vi "Main.vi"() -> ()   [LabVIEW 2020]
uses:
  NI-9361 (C Series)/NI-9361 (C Series).lvclass
  C:/Users/Thomas/Documents/YouTube Videos/Interfaces/Interface HAL Example/C-Series/C-Series.lvclass
  NI-9421 (C Series)/NI-9421 (C Series).lvclass
  C:/Users/Thomas/Documents/YouTube Videos/Interfaces/Interface HAL Example/DIO/DIO.lvclass
  C-Series/C-Series.lvclass
  NI-6537 (PXIe)/NI-6537 (PXIe).lvclass
  C:/Users/Thomas/Documents/YouTube Videos/Interfaces/Interface HAL Example/PXIe/PXIe.lvclass
  PXIe/PXIe.lvclass
  Voltage Input/Voltage Input.lvclass
  NI-6115 (PXIe-6368)/NI-6368 (PXIe).lvclass
  C:/Users/Thomas/Documents/YouTube Videos/Interfaces/Interface HAL Example/Voltage Input/Voltage Input.lvclass
  C:/Users/Thomas/Documents/YouTube Videos/Interfaces/Interface HAL Example/DMM/Multifunction IO.lvclass
  NI-9381 (c series)/NI-9381 (c series).lvclass
  NI-9239 (C Series)/NI-9239 (C Series).lvclass
  PSU/AIO.lvclass
  Counter/Counter.lvclass
  DIO/DIO.lvclass
  Hardware/Instrument.lvclass
  DMM/Multifunction IO.lvclass
panel:
  in  "Select":bool
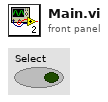
[diagram p1: front panel]
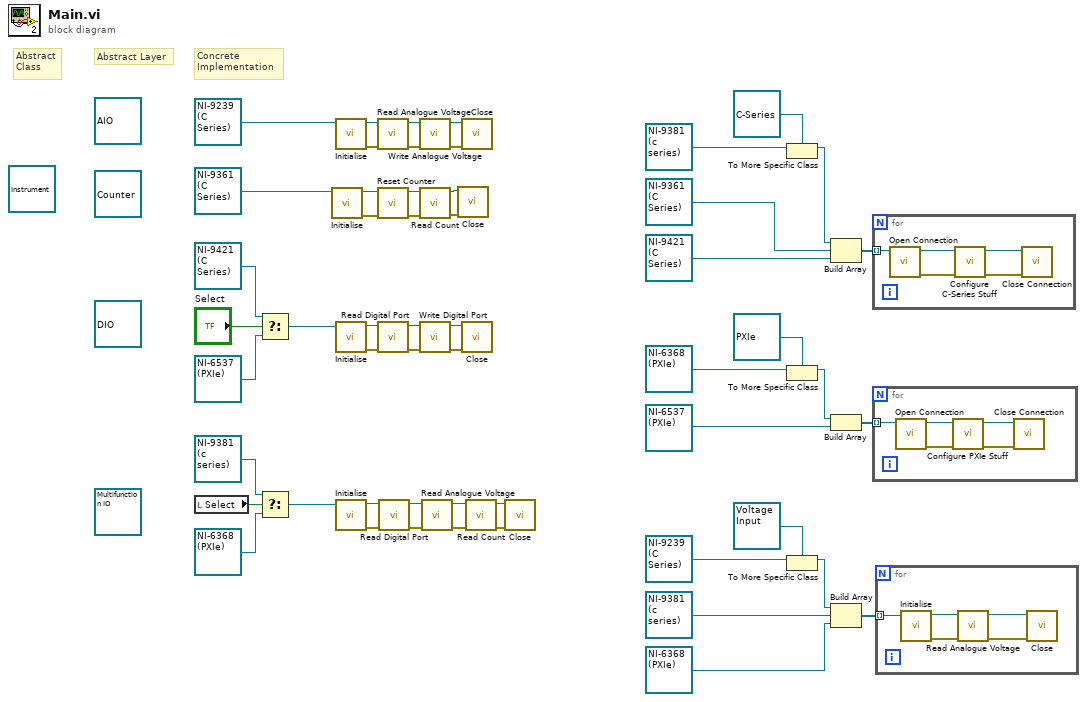
[diagram p0: block diagram]
diagram:
  (unwired) refnum<class "Multifunction IO.lvclass"> refnum ("Multifunction IO.lvclass")
  (unwired) refnum<class "Instrument.lvclass"> refnum ("Instrument.lvclass")
  (unwired) refnum<class "DIO.lvclass"> refnum ("DIO.lvclass")
  (unwired) refnum<class "Counter.lvclass"> refnum ("Counter.lvclass")
  (unwired) refnum<class "AIO.lvclass"> refnum ("AIO.lvclass")
  # "Concrete\nImplementation"
  # "Abstract\nClass"
  # "Abstract Layer"
  n1 = local read "Select"() -> (w34:bool)
  n2 = Select(t=refnum<class "NI-9421 (C Series).lvclass"> refnum ("NI-9421 (C Series).lvclass"), s="Select", f=refnum<class "NI-6537 (PXIe).lvclass"> refnum ("NI-6537 (PXIe).lvclass")) -> (s? t:f=w36:refnum<class "DIO.lvclass">)
  n3 = Select(t=refnum<class "NI-9381 (c series).lvclass"> refnum ("NI-9381 (c series).lvclass"), s=w34, f=refnum<class "NI-6368 (PXIe).lvclass"> refnum ("NI-6368 (PXIe).lvclass")) -> (s? t:f=w31:refnum<class "Multifunction IO.lvclass">)
  n4 = call-dynamic "Initialise.vi"("Instrument in"=refnum<class "NI-9361 (C Series).lvclass"> refnum ("NI-9361 (C Series).lvclass")) -> ("error out"=w23:errorcluster, "Instrument out"=w24:refnum<class "NI-9361 (C Series).lvclass">)  [unwired: 9 in]
  n5 = call-dynamic "Initialise.vi"("Instrument in"=refnum<class "NI-9239 (C Series).lvclass"> refnum ("NI-9239.lvclass")) -> ("error out"=w48:errorcluster, "Instrument out"=w51:refnum<class "NI-9239 (C Series).lvclass">)  [unwired: 9 in]
  n6 = call-dynamic "Initialise.vi"("Instrument in"=w36) -> ("error out"=w45:errorcluster, "Instrument out"=w44:refnum<class "DIO.lvclass">)  [unwired: 9 in]
  n7 = call-dynamic "Initialise.vi"("Instrument in"=w31) -> ("error out"=w3:errorcluster, "Instrument out"=w6:refnum<class "Multifunction IO.lvclass">)  [unwired: 9 in]
  n8 = call-dynamic "Read Analogue Voltage.vi"("error in (no error)"=w48, "AIO in"=w51) -> ("error out"=w49:errorcluster, "AIO out"=w52:refnum<class "NI-9239 (C Series).lvclass">)  [unwired: 8 in]
  n9 = call-dynamic "Reset Counter.vi"("error in (no error)"=w23, "Counter in"=w24) -> ("error out"=w46:errorcluster, "Counter out"=w47:refnum<class "NI-9361 (C Series).lvclass">)  [unwired: 8 in]
  n10 = call-dynamic "Read Digital Port.vi"("error in (no error)"=w45, "DIO in"=w44) -> ("error out"=w40:errorcluster, "DIO out"=w43:refnum<class "DIO.lvclass">)  [unwired: 8 in]
  n11 = call-dynamic "Read Digital Port.vi"("error in (no error)"=w3, "Multifunction IO in"=w6) -> ("error out"=w4:errorcluster, "Multifunction IO out"=w7:refnum<class "Multifunction IO.lvclass">)  [unwired: 8 in]
  n12 = call-dynamic "Write Analogue Voltage.vi"("error in (no error)"=w49, "AIO in"=w52) -> ("error out"=w50:errorcluster, "AIO out"=w53:refnum<class "NI-9239 (C Series).lvclass">)  [unwired: 8 in]
  n13 = call-dynamic "Read Count.vi"("error in (no error)"=w46, "Counter in"=w47) -> ("error out"=w26:errorcluster, "Counter out"=w25:refnum<class "NI-9361 (C Series).lvclass">)  [unwired: 8 in]
  n14 = call-dynamic "Write Digital Port.vi"("error in (no error)"=w40, "DIO in"=w43) -> ("error out"=w41:errorcluster, "DIO out"=w42:refnum<class "DIO.lvclass">)  [unwired: 8 in]
  n15 = call-dynamic "Read Analogue Voltage.vi"("error in (no error)"=w4, "Multifunction IO in"=w7) -> ("error out"=w5:errorcluster, "Multifunction IO out"=w8:refnum<class "Multifunction IO.lvclass">)  [unwired: 8 in]
  n16 = call-dynamic "Close.vi"("error in (no error)"=w26, "Instrument in"=w25) -> ()  [unwired: 8 in, 2 out]
  n17 = call-dynamic "Close.vi"("error in (no error)"=w50, "Instrument in"=w53) -> ()  [unwired: 8 in, 2 out]
  n18 = call-dynamic "Close.vi"("error in (no error)"=w41, "Instrument in"=w42) -> ()  [unwired: 8 in, 2 out]
  n19 = call-dynamic "Read Count.vi"("error in (no error)"=w5, "Multifunction IO in"=w8) -> ("error out"=w2:errorcluster, "Multifunction IO out"=w1:refnum<class "Multifunction IO.lvclass">)  [unwired: 8 in]
  n20 = call-dynamic "Close.vi"("error in (no error)"=w2, "Instrument in"=w1) -> ()  [unwired: 8 in, 2 out]
  n21 = To More Specific Class(target class=refnum<class "C-Series.lvclass"> refnum ("C-Series.lvclass"), reference=refnum<class "NI-9381 (c series).lvclass"> refnum ("NI-9381 (c series).lvclass")) -> (specific class reference=w21:refnum<class "C-Series.lvclass">)  [unwired: 1 in, 1 out]
  n22 = To More Specific Class(target class=refnum<class "PXIe.lvclass"> refnum ("PXIe.lvclass"), reference=refnum<class "NI-6368 (PXIe).lvclass"> refnum ("NI-6368 (PXIe).lvclass")) -> (specific class reference=w16:refnum<class "PXIe.lvclass">)  [unwired: 1 in, 1 out]
  n23 = To More Specific Class(target class=refnum<class "Voltage Input.lvclass"> refnum ("Voltage Input.lvclass"), reference=refnum<class "NI-9239 (C Series).lvclass"> refnum ("NI-9239.lvclass")) -> (specific class reference=w12:refnum<class "Voltage Input.lvclass">)  [unwired: 1 in, 1 out]
  n24 = Build Array(w21, refnum<class "NI-9361 (C Series).lvclass"> refnum ("NI-9361 (C Series).lvclass"), refnum<class "NI-9421 (C Series).lvclass"> refnum ("NI-9421 (C Series).lvclass")) -> (w28:refnum<class "C-Series.lvclass">[])
  n25 = Build Array(w16, refnum<class "NI-6537 (PXIe).lvclass"> refnum ("NI-6537 (PXIe).lvclass")) -> (w19:refnum<class "PXIe.lvclass">[])
  n26 = Build Array(w12, refnum<class "NI-9381 (c series).lvclass"> refnum ("NI-9381 (c series).lvclass"), refnum<class "NI-6368 (PXIe).lvclass"> refnum ("NI-6368 (PXIe).lvclass")) -> (w9:refnum<class "Voltage Input.lvclass">[])
  n27 = for {
    tunnel: w28 -> [w54] mode=indexing
    n28 = call-dynamic "Open Connection.vi"("Chassis in"=w54) -> ("error out"=w55:errorcluster, "Chassis out"=w56:refnum<class "C-Series.lvclass">)  [unwired: 9 in]
    n29 = call-dynamic "Configure C-Series Stuff.vi"("error in (no error)"=w55, "C-Series in"=w56) -> ("error out"=w57:errorcluster, "C-Series out"=w58:refnum<class "C-Series.lvclass">)  [unwired: 8 in]
    n30 = call-dynamic "Close Connection.vi"("error in (no error)"=w57, "Chassis in"=w58) -> ()  [unwired: 8 in, 2 out]
  }
  n31 = for {
    tunnel: w19 -> [w63] mode=indexing
    n32 = call-dynamic "Open Connection.vi"("Chassis in"=w63) -> ("error out"=w61:errorcluster, "Chassis out"=w62:refnum<class "PXIe.lvclass">)  [unwired: 9 in]
    n33 = call-dynamic "Configure PXIe Stuff.vi"("error in (no error)"=w61, "PXIe in"=w62) -> ("error out"=w60:errorcluster, "PXIe out"=w59:refnum<class "PXIe.lvclass">)  [unwired: 8 in]
    n34 = call-dynamic "Close Connection.vi"("error in (no error)"=w60, "Chassis in"=w59) -> ()  [unwired: 8 in, 2 out]
  }
  n35 = for {
    tunnel: w9 -> [w68] mode=indexing
    n36 = call-dynamic "Initialise.vi"("DAQ in"=w68) -> ("error out"=w66:errorcluster, "DAQ out"=w67:refnum<class "Voltage Input.lvclass">)  [unwired: 9 in]
    n37 = call-dynamic "Read Analogue Voltage.vi"("error in (no error)"=w66, "Voltage Input in"=w67) -> ("error out"=w65:errorcluster, "Voltage Input out"=w64:refnum<class "Voltage Input.lvclass">)  [unwired: 8 in]
    n38 = call-dynamic "Close.vi"("error in (no error)"=w65, "DAQ in"=w64) -> ()  [unwired: 8 in, 2 out]
  }
